vi "Auto settings.vi"(8 "error in (no error)":errorcluster, 10 "Array":dbl[](array[numeric]), 11 "Pick Up Tool Fixture in":refnum<class "Pick Up Tool Fixture.lvclass">) -> (0 "error out":errorcluster, 3 "Pick Up Tool Fixture out":refnum<class "Pick Up Tool Fixture.lvclass">)   [LabVIEW 2020, in "Pick Up Tool Fixture.lvclass"]
uses:
  Pick Up Tool Fixture.lvclass
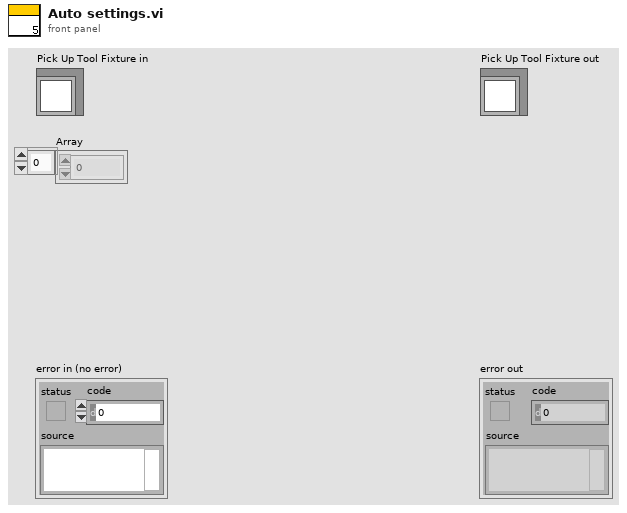
[diagram p1: front panel]
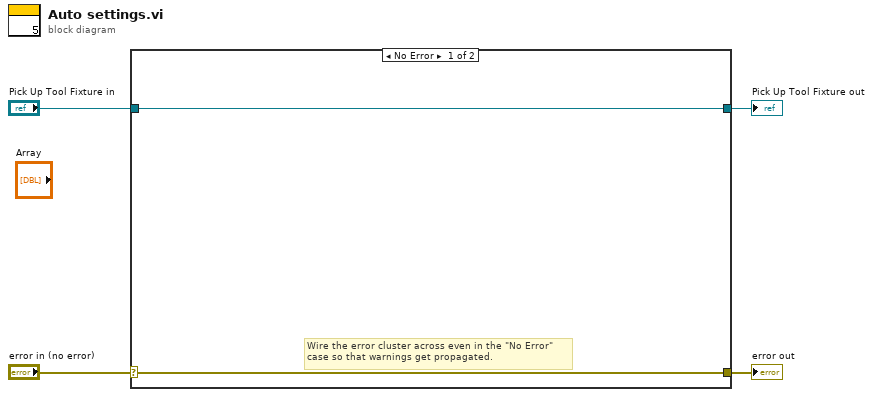
[diagram p0: block diagram]
diagram:
  n1 = case shown="No Error" "error in (no error)" {
    selector: "error in (no error)" -> [w5 w8]
    tunnel: [w5 w8] -> w3
    tunnel: [w6 w7] -> w1
    tunnel: "Pick Up Tool Fixture in" -> [w6 w7]
    frame No Error {
      # "Wire the error cluster across even in the \"No Error\"\ncase so that warnings get propagated."
    }
    frame Error {
    }
  }
  "error out" <- w3
  "Pick Up Tool Fixture out" <- w1
